vi "Register Group.vi"(8 "error in (no error)":errorcluster, 10 "Group":refnum<class "GroupAbstract.lvclass">, 11 "Task in":refnum<class "Task.lvclass">) -> (0 "error out":errorcluster, 3 "Task out":refnum<class "Task.lvclass">)   [LabVIEW 2020, in "Volatus.lvlib" / "Task.lvclass"]
uses:
  Task.lvclass
  Task.lvclass/Task.ctl
  lv-vecto/Vecto/GroupAbstract/GroupAbstract.lvclass
  <vilib>/Utility/miscctls.llb/LVMapReplaceAction.ctl
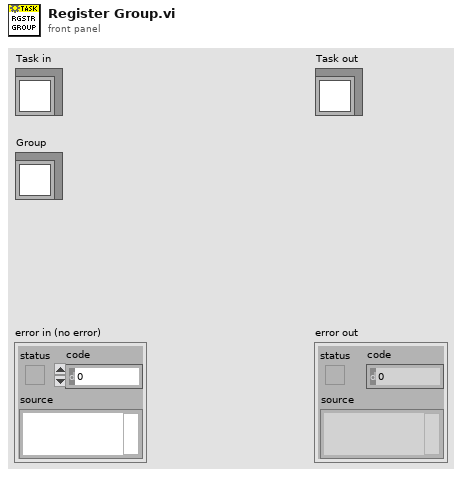
[diagram p1: front panel]
types:
  T1 = typedef "LVMapReplaceAction.ctl" = enum32{"Modify Entry only if found", "Add or Modify Entry", "Delete Entry"}
  T2 = map{string, refnum<class "GroupAbstract.lvclass">}
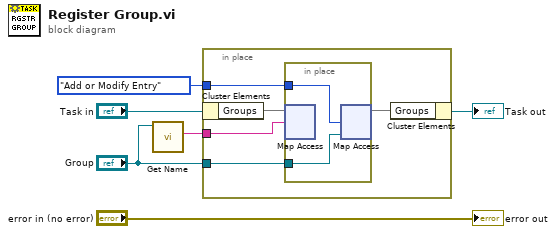
[diagram p0: block diagram]
diagram:
  n1 = call "Get Name.vi"("GroupAbstract in"="Group") -> ("Name"=w4:string)  [unwired: 8 in, 2 out]
  n2 = in-place {
    in-place-border: w4 -> [w10]
    in-place-border: "Group" -> [w9]
    in-place-border: LVMapReplaceAction."Add or Modify Entry" ("action") -> [w8]
    n3 = in-place-cluster #1("Task in") -> ("Groups"=w11:T2)
    n4 = in-place {
      in-place-border: w9 -> [w13]
      in-place-border: w8 -> [w12]
      n5 = in-place-map #2(w11, w10) -> ()  [unwired: 1 in, 2 out]
      n6 = in-place-map #2(w13, w12) -> (w7:T2)  [unwired: 2 out]
    }
    n7 = in-place-cluster #1("Groups"=w7) -> (→"Task out":refnum<class "Task.lvclass">)
  }
  "error out" <- "error in (no error)"
